vi "SuperSimpleMotorTest.vi"() -> ()   [LabVIEW 2009]
uses:
  <vilib>/Platform/TimedLoop/XDataNode/XDataNode.xnode
  <vilib>/Platform/TimedLoop/XDataNode/loadlvalarms.vi
  <vilib>/Platform/TimedLoop/XDataNode/timing_clust.ctl
  <vilib>/Platform/TimedLoop/XDataNode/nitl_modes.ctl
  <vilib>/Platform/TimedLoop/XDataNode/wakeup.ctl
  <vilib>/eio/EIONode/EIONode.xnode
  <vilib>/rvi/eio/nirviEIOImplementation/nirviEIOImplementation.xnode
  <vilib>/rvi/eio/common/nirviEmuTemplateMethod_noerrors.vi
  <vilib>/rvi/eio/common/nirviEmuClasses.ctl
  <vilib>/Platform/TimedLoop/XDataNode/XDNodeRunTimeDep.lvlib
panel:
  in  "stop":bool
  in  "M2 Enable":bool
  in  "M1 Enable":bool
  in  "M0 Enable":bool
  in  "M2 output":fxp<+/-,20,5>
  in  "M1 output":fxp<+/-,20,5>
  in  "M0 output":fxp<+/-,20,5>
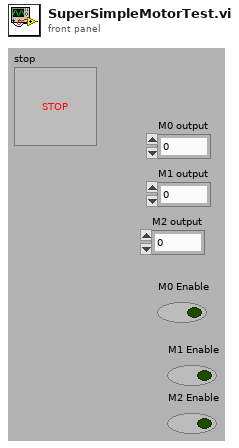
[diagram p1: front panel]
types:
  T1 = typedef "XDNodeRunTimeDep.lvlib/timing_clust.ctl" = cluster{"Expected End [f-1]":u64, "Actual End [f-1]":u64, "Finished Late? [f-1]":bool, "Expected End [i-1]":u64, "Actual End [i-1]":u64, "Finished Late? [i-1]":bool, "Expected Start [i]":u64, "Actual Start [i]":u64, "Expected Start [f]":u64, "Actual Start [f]":u64, "Source Name":string, "Structure Name":string, "Period":i64, "Deadline":i64, "Offset":i64, "Start":i64, "Priority":i32, "Timeout":i32, "Mode":T2, "Wakeup Reason":T3, "Error":errorcluster, "Source Type":string, "Secondary Source Type":string, "Global End Time":u64, "Global Start Time":u64, "Frame Duration":u64, "Iteration Duration":u64, "Assigned CPU":i32, "I/O Scan Engine Mode":u32}
  T2 = typedef "XDNodeRunTimeDep.lvlib/nitl_modes.ctl" = enum32{"No Change", "Process missed periods, maintain original phase", "Discard missed periods, maintain original phase", "Process missed periods, ignore original phase", "Discard missed periods, ignore original phase"}
  T3 = typedef "XDNodeRunTimeDep.lvlib/wakeup.ctl" = enum32{"Normal", "Aborted", "Asynchronous wakeup", "Timing source error", "Timed loop error", "Timeout"}
  T4 = typedef "nirviEmuClasses.ctl" = enum16{"IO Read", "IO Write", "Method", "Property Read", "Property Write"}
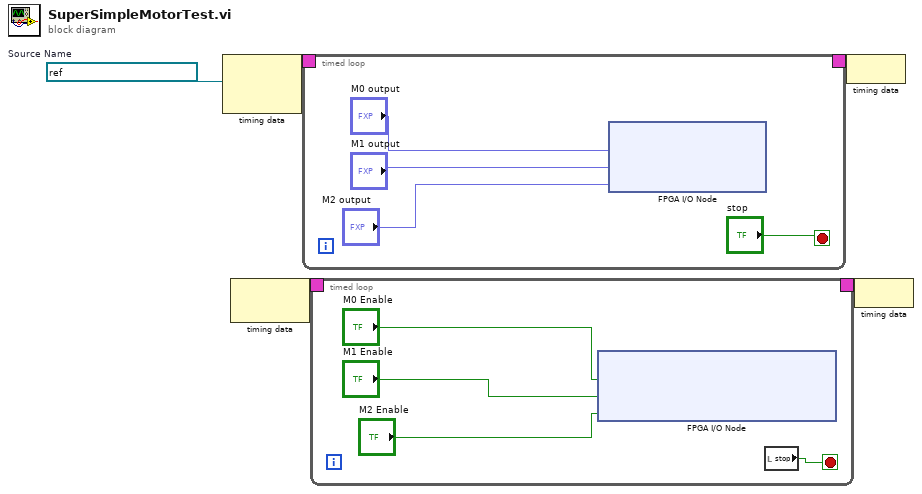
[diagram p0: block diagram]
diagram:
  w1 = refnum<k21> "40 MHz Onboard Clock"  # Source Name
  n1 = node-c288(w1) -> (w3:T1)  [unwired: 1 in]
  n2 = node-c288() -> (w5:T1)  [unwired: 1 in]
  n3 = timed-loop {
    timing: w3 -> [_]
    timing-out: [_] -> w2
    stop <- "stop" stop-if-true
    n4 = xnode "FPGA I/O Node"("Drive Motor Speed"="M0 output", "Steering Motor Speed"="M1 output", "Lidar Motor Speed"="M2 output") -> ()  [unwired: 3 in, 3 out]
  }
  n5 = timed-loop {
    timing: w5 -> [_]
    timing-out: [_] -> w4
    stop <- w45 stop-if-true
    n6 = xnode "FPGA I/O Node"("Drive Motor Inhibit (Non-Functional)"="M0 Enable", "Steering Motor Inhibit"="M1 Enable", "Lidar Motor Inhibit"="M2 Enable") -> ()  [unwired: 3 in, 3 out]
    n7 = local read "stop"() -> (w45:bool)
  }
  n8 = node-c288(w2) -> ()
  n9 = node-c288(w4) -> ()
